vi "WS1050_RFFE_ST Scope Single Bit Measurement Debug Ver1.1.vi"(0 "RFFE PIC":refnum<visa-resource-name>="COM7", 1 "A3643A GPIB":refnum<visa-resource-name>="GPIB1::6::INSTR", 3 "LOT#":string="444AB", 4 "WAFER#":string="04", 5 "DUT SN":string="SN01", 7 "error in (no error)":errorcluster, 8 "Scope USB":refnum<visa-resource-name>="USB0::0x0699::0x0405::C010240::INSTR", 9 "GROUP":string, 12 "path":path=path "C:/Andy/WS1050/ST Test/Debug Ver1.1", 14 "Start":bool, 15 "Stop Loop":bool, 16 "Initilize RFFE ?":bool=TRUE, 17 "stop":bool, 20 "Scope \nSet Up":bool, 22 "Comment":string) -> (18 "ST Data Out":string[](array[string])=["824.709800E-9", "99.100000E+36", "14.400000E-3", "99.100000E+36", "687.070300E-9", "14.000000E-3", "991.902900E-9", "99.100000E+36", "30.800000E-3", "99.100000E+36", "729.561600E-9", "28.400000E-3", "794.023400E-9", "99.100000E+36", "66.000000E-3", "99.100000E+36", "698.320300E-9", "64.000000E-3", "677.011700E-9", "99.100000E+36", "172.000000E-3", "99.100000E+36", "781.972700E-9", "168.000000E-3", "1.047500E-6", "99.100000E+36", "252.000000E-3", "99.100000E+36", "806.324900E-9", "248.000000E-3", "1.166000E-6", "99.100000E+36", "384.000000E-3", "99.100000E+36", "800.507800E-9", "372.000000E-3", "3.559500E-6", "99.100000E+36", "536.000000E-3", "99.100000E+36", "804.648400E-9", "512.000000E-3", "2.976000E-6", "99.100000E+36", "664.000000E-3", "99.100000E+36", "794.980500E-9", "640.000000E-3", "1.596500E-6", "99.100000E+36", "792.000000E-3", "99.100000E+36", "835.996100E-9", "768.000000E-3", "3.144000E-6", "99.100000E+36", "912.000000E-3", "99.100000E+36", "849.980500E-9", "880.000000E-3", "1.416700E-6", "99.100000E+36", "1.000000E+0", "99.100000E+36", "864.023400E-9", "960.000000E-3", "1.295500E-6", "99.100000E+36", "1.060000E+0", "99.100000E+36", "858.515600E-9", "1.020000E+0", "1.204000E-6", "99.100000E+36", "1.080000E+0", "99.100000E+36", "934.023400E-9", "1.060000E+0", "1.336000E-6", "99.100000E+36", "1.140000E+0", "99.100000E+36", "1.063300E-6", "1.100000E+0", "1.338000E-6", "99.100000E+36", "1.160000E+0", "99.100000E+36", "1.149500E-6", "1.140000E+0", "1.280000E-6", "99.100000E+36", "1.200000E+0", "99.100000E+36", "1.149300E-6", "1.160000E+0", "1.380000E-6", "99.100000E+36", "1.200000E+0", "99.100000E+36", "1.173000E-6", "1.160000E+0", "1.408000E-6", "99.100000E+36", "1.220000E+0", "99.100000E+36", "1.194000E-6", "1.180000E+0", "1.215000E-6", "99.100000E+36", "70.000000E-3", "99.100000E+36", "1.033300E-6", "68.000000E-3", "2.179200E-6", "99.100000E+36", "170.000000E-3", "99.100000E+36", "1.326500E-6", "158.000000E-3", "1.427300E-6", "99.100000E+36", "316.000000E-3", "99.100000E+36", "1.133000E-6", "308.000000E-3", "1.174000E-6", "99.100000E+36", "680.000000E-3", "99.100000E+36", "915.325500E-9", "620.000000E-3", "1.356000E-6", "99.100000E+36", "920.000000E-3", "99.100000E+36", "1.156000E-6", "880.000000E-3", "1.310000E-6", "99.100000E+36", "960.000000E-3", "99.100000E+36", "1.476500E-6", "980.000000E-3", "1.482000E-6", "99.100000E+36", "1.080000E+0", "99.100000E+36", "1.526000E-6", "1.060000E+0", "1.539500E-6", "99.100000E+36", "1.140000E+0", "99.100000E+36", "1.666000E-6", "1.120000E+0", "1.567000E-6", "99.100000E+36", "1.160000E+0", "99.100000E+36", "1.768000E-6", "1.160000E+0", "1.520000E-6", "99.100000E+36", "1.200000E+0", "99.100000E+36", "1.804000E-6", "1.160000E+0", "1.515000E-6", "99.100000E+36", "1.200000E+0", "99.100000E+36", "1.898000E-6", "1.180000E+0", "1.498000E-6", "99.100000E+36", "1.220000E+0", "99.100000E+36", "1.858000E-6", "1.220000E+0", "1.449000E-6", "99.100000E+36", "1.220000E+0", "99.100000E+36", "1.870000E-6", "1.200000E+0", "1.458500E-6", "99.100000E+36", "1.220000E+0", "99.100000E+36", "1.860000E-6", "1.200000E+0", "1.428500E-6", "99.100000E+36", "1.220000E+0", "99.100000E+36", "1.870000E-6", "1.200000E+0", "1.350000E-6", "99.100000E+36", "1.200000E+0", "99.100000E+36", "1.918500E-6", "1.220000E+0", "1.468500E-6", "99.100000E+36", "1.220000E+0", "99.100000E+36", "1.938700E-6", "1.220000E+0", "1.390000E-6", "99.100000E+36", "1.200000E+0", "99.100000E+36", "1.917500E-6", "1.200000E+0", "634.023400E-9", "99.100000E+36", "46.000000E-3", "99.100000E+36", "1.470000E-6", "40.000000E-3", "1.126000E-6", "99.100000E+36", "84.000000E-3", "99.100000E+36", "1.137000E-6", "84.000000E-3", "1.103700E-6", "99.100000E+36", "238.000000E-3", "99.100000E+36", "1.126200E-6", "226.000000E-3", "1.091000E-6", "99.100000E+36", "512.000000E-3", "99.100000E+36", "1.010000E-6", "480.000000E-3", "3.414000E-6", "99.100000E+36", "760.000000E-3", "99.100000E+36", "949.980500E-9", "700.000000E-3", "1.376000E-6", "99.100000E+36", "940.000000E-3", "99.100000E+36", "1.268000E-6", "920.000000E-3", "1.268000E-6", "99.100000E+36", "1.020000E+0", "99.100000E+36", "1.278000E-6", "980.000000E-3", "1.294000E-6", "99.100000E+36", "1.060000E+0", "99.100000E+36", "1.334000E-6", "1.060000E+0", "1.488000E-6", "99.100000E+36", "1.160000E+0", "99.100000E+36", "1.448000E-6", "1.120000E+0", "1.515000E-6", "99.100000E+36", "1.200000E+0", "99.100000E+36", "1.534000E-6", "1.160000E+0", "1.516000E-6", "99.100000E+36", "1.240000E+0", "99.100000E+36", "1.628000E-6", "1.220000E+0", "1.602000E-6", "99.100000E+36", "1.280000E+0", "99.100000E+36", "1.557000E-6", "1.240000E+0", "1.610000E-6", "99.100000E+36", "1.300000E+0", "99.100000E+36", "1.637500E-6", "1.260000E+0", "1.580000E-6", "99.100000E+36", "1.300000E+0", "99.100000E+36", "1.724000E-6", "1.280000E+0", "1.611000E-6", "99.100000E+36", "1.320000E+0", "99.100000E+36", "1.722000E-6", "1.280000E+0", "1.611000E-6", "99.100000E+36", "1.320000E+0", "99.100000E+36", "1.770000E-6", "1.300000E+0", "1.608000E-6", "99.100000E+36", "1.320000E+0", "99.100000E+36", "1.780000E-6", "1.300000E+0", "1.601000E-6", "99.100000E+36", "1.320000E+0", "99.100000E+36", "1.795000E-6", "1.300000E+0"], 19 "ST Header Out":string[](array[string]), 21 "Status":string="Idle....", 27 "error out":errorcluster)   [LabVIEW 2012]
doc: "Ver1.0 has calculated and recorded both 60% and 95% of the AMP"
uses:
  <instrlib>/Tektronix DPO MSO 2000 4000 Series/Tektronix DPO MSO 2000 4000 Series.lvlib
panel:
  out "Filtered Signal":dbl[](graph)
  out "Signal":dbl[](graph)
  in  "% Amp_T3":dbl=0.95
  in  "% Amp_T2":dbl=0.9
  in  "Debug":bool
  in  "Loop Delay(s)":u32
  out "Index":i32
  in  "% Amp_T1":dbl=0.6
  out "Cmd Out":string
  in  "Bandwidth":u16(ring)=3 items=["FULL", "250 MHz", "150 MHz", "20 MHz"]
  out "Test Program Name":string=" WS1050 ST Scope SBM Debug Ver1.1"
  out "dt":dbl=1e-08
  in  "Timebase":dbl=0.0001
  in  "RFFE Action":i32(ring)=2 items=["-", "Charge Pump Off", "Charge Pump On", "-", "DVA OFF", "DVA ON", "Charge Pump to 40V", "Charge Pump to 35V", "Trim Code 26", "Trim Code 30", "Trim Code 32", "Trim Code 33", "Trim Code 42", "Trim Code 44", "Trim Code 46", "Trim Code 48", "Trim Code 49", "Trim Code 50", "All Drivers Off", "All Drivers On", "Reg1 On", "Reg2 On", "Reg3 On", "Reg4 On"]
  in  "RFFE Action":bool
  in  "Closing Cheetah function calls":i32(listbox)
  # "Updated based on Debug\n\n 1.  Updated WS1050 Extract Data From Scope_ST_CLK SubVI by adding another point   calculated based on 95% of Amp and 1 us for the CLK starts from 21st"
  # "Company:  WiSpry Inc\n20 Fairbanks Ste 198, Irvine\n\nAuthor:  Andy V Tran\nDate:  07/08/2015\nTP:  ST Scope Single Bit"
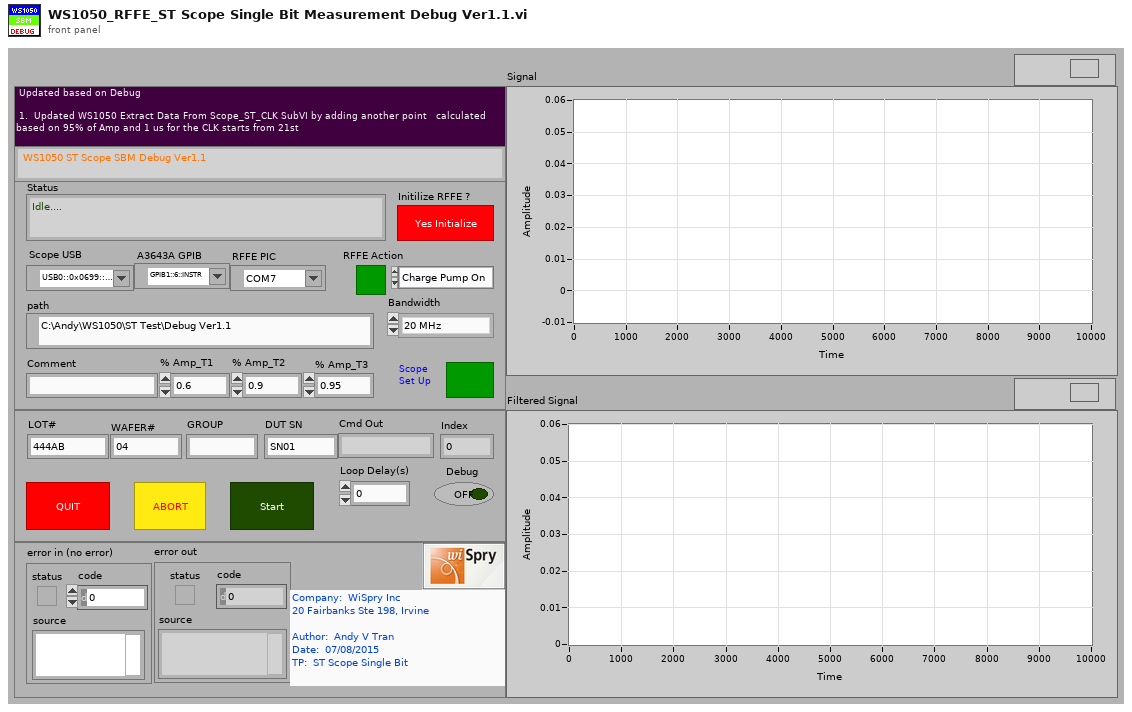
[diagram p1: front panel]
types:
  T1 = enum16{"open", "replace", "create", "open or create", "replace or create", "replace or create with confirmation"}
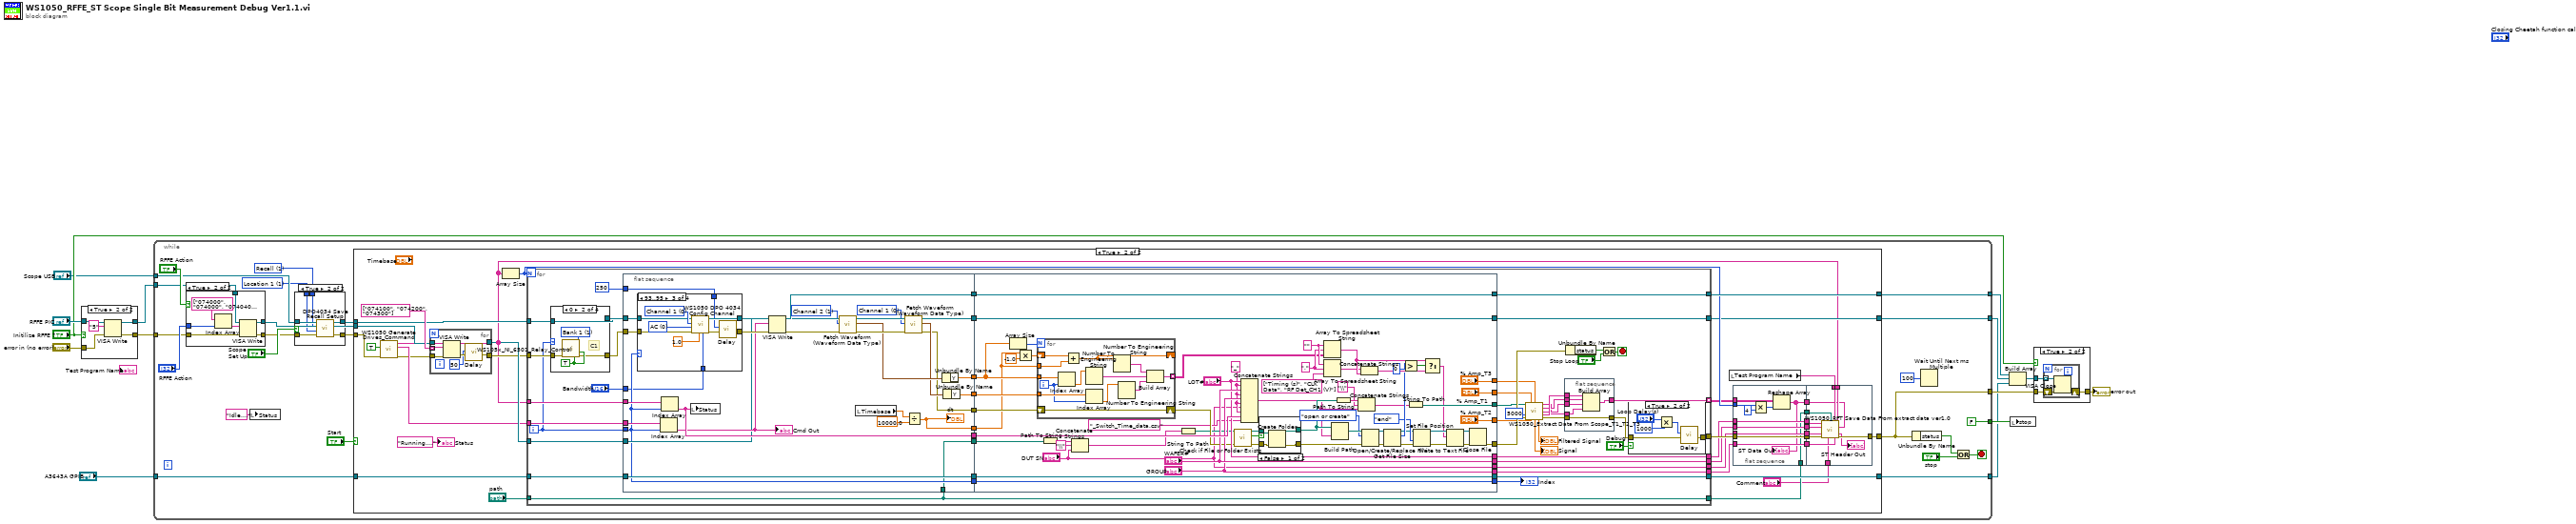
[diagram p0: block diagram]
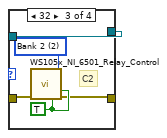
[diagram p7: hidden frame]
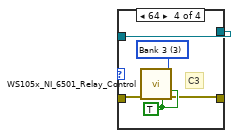
[diagram p8: hidden frame]
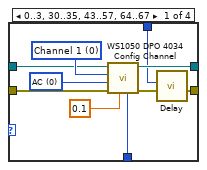
[diagram p9: hidden frame]
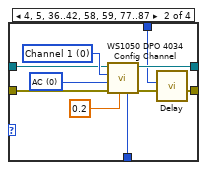
[diagram p10: hidden frame]
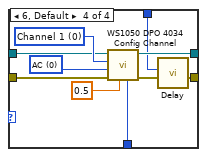
[diagram p11: hidden frame]
diagram:
  n1 = case shown="True" "Initilize RFFE ?" {
    tunnel: [w16 w18] -> w7
    tunnel: "error in (no error)" -> [w16 w19]
    tunnel: "RFFE PIC" -> [w15 w21]
    tunnel: [w15 w17] -> w9
    frame False {
    }
    frame True {
      n2 = VISA Write(VISA resource name=w21, write buffer="5", error in (no error)=w19) -> (VISA resource name out=w17:refnum<visa-resource-name>, error out=w18:errorcluster)  [unwired: 1 out]
    }
  }
  n3 = while {
    tunnel: [w37] -> w11
    tunnel: w7 -> [w30]
    tunnel: "A3643A GPIB" -> [w38]
    tunnel: [w36] -> w2
    tunnel: w9 -> [w29]
    tunnel: [w31] -> w4
    tunnel: [w27] -> w3
    tunnel: "Scope USB" -> [w26]
    tunnel: [FALSE ("stop")] -> w5
    stop <- w45 stop-if-true
    w23 = u16 1 items=["Location 1"=1, "Location 2"=2, "Location 3"=3, "Location 4"=4, "Location 5"=5, "Location 6"=6, "Location 7"=7, "Location 8"=8, "Location 9"=9, "Location 10"=10] ("Memory Location (1: Location 1)")
    w24 = u16 1 items=["Save", "Recall"] ("Operation (0: Save)")
    n4 = case shown="True" "RFFE Action" {
      tunnel: "RFFE Action" -> [_ w62]
      tunnel: w30 -> [w54 w60]
      tunnel: w29 -> [w55 w59]
      tunnel: [w55 w58] -> w28
      tunnel: [w54 w56] -> w25
      frame False {
      }
      frame True {
        n5 = Index Array(array=string[] ["074000", "074000", "074040", "", "074820", "074800", "074776", "07476F"], index=w62) -> (element=w57:string)
        n6 = VISA Write(VISA resource name=w59, write buffer=w57, error in (no error)=w60) -> (VISA resource name out=w58:refnum<visa-resource-name>, error out=w56:errorcluster)  [unwired: 1 out]
      }
    }
    n7 = local write "Status"("Idle...." ("Status")) -> ()
    n8 = case shown="True" "Scope \nSet Up" {
      tunnel: w25 -> [w47 w53]
      tunnel: [w47 w52] -> w33
      tunnel: w26 -> [w46 w51]
      tunnel: [w46 w50] -> w34
      tunnel: w24 -> [_ w49]
      tunnel: w23 -> [_ w48]
      frame False {
      }
      frame True {
        n9 = call "DPO4034 Save Recall Setup.vi"("error in (no error)"=w53, "Save/Recall"=w48, "Location"=w49, "VISA resource name"=w51) -> ("error out"=w52:errorcluster, "VISA resource name out"=w50:refnum<visa-resource-name>)  [unwired: 6 in]
      }
    }
    n10 = case shown="True" "Start" {
      tunnel: [w66 w83] -> w27
      tunnel: w34 -> [w66 w82]
      tunnel: w33 -> [w65 w71]
      tunnel: w38 -> [w64 w84]
      tunnel: [w64 w98] -> w36
      tunnel: [w65 w96] -> w37
      tunnel: [w63 w90] -> w31
      tunnel: w28 -> [w63 w86]
      frame False {
      }
      frame True {
        n11 = call "WS1050 Generate Drives_Command.vi"("error in (no error)"=w71, "ALL/UP-DN"=TRUE) -> ("error out"=w70:errorcluster, "Cmd"=w72:string[], "Driver Name"=w73:string[])  [unwired: 7 in]
        n12 = for {
          tunnel: w70 -> [w130]
          tunnel: w86 -> [w129]
          tunnel: [w128] -> w89
          tunnel: [w126] -> w88
          tunnel: string[] ["074100", "074200", "074300"] -> [w127] mode=indexing
          n13 = VISA Write(VISA resource name=w129, write buffer=w127, error in (no error)=w130) -> (VISA resource name out=w128:refnum<visa-resource-name>, error out=w125:errorcluster)  [unwired: 1 out]
          n14 = call "Delay.vi"("error in (no error)"=w125, "milliseconds to wait"=u32 50) -> ("error out"=w126:errorcluster)  [unwired: 9 in]
        }
        n15 = Array Size(array=w73) -> (size(s)=w85:i32)
        n16 = for {
          N: w85 -> [_]
          tunnel: [w143] -> w97
          tunnel: "path" -> [w148]
          tunnel: w84 -> [w172]
          tunnel: [w170] -> w98
          tunnel: w88 -> [w166]
          tunnel: w73 -> [w169]
          tunnel: w72 -> [w167]
          tunnel: [w163] -> w95
          tunnel: [w162] -> w94
          tunnel: [w161] -> w93
          tunnel: [w160] -> w92
          tunnel: w89 -> [w159]
          tunnel: [w157] -> w90
          tunnel: [w156] -> w83
          tunnel: w82 -> [w155]
          tunnel: [w148] -> w75
          tunnel: [w151] -> w69 mode=indexing
          i -> [w154]
          stop <- w178 stop-if-true
          n17 = case shown="0" w154 {
            tunnel: w166 -> [w193 w199 w204 w209]
            tunnel: [w193 w195 w200 w205] -> w165
            tunnel: w155 -> [w194 w196 w201 w206]
            tunnel: [w194 w196 w201 w206] -> w164
            frame 1, Default {
            }
            frame 0 {
              w197 = TRUE ("Relay_ 10")
              w198 = u16 1 items=["All Off", "Bank 1", "Bank 2", "Bank 3"] ("Ring")
              # "C1"
              n18 = call "WS105x_NI_6501_Relay_Control.vi"("Ring"=w198, "Relay_ 11"=w197, "error in (no error)"=w199, "Relay_ 10"=w197) -> ("error out"=w195:errorcluster)  [unwired: 2 in, 9 out]
            }
            frame 32 {
              w202 = TRUE ("Relay_ 10")
              w203 = u16 2 items=["All Off", "Bank 1", "Bank 2", "Bank 3"] ("Ring")
              # "C2"
              n19 = call "WS105x_NI_6501_Relay_Control.vi"("Ring"=w203, "Relay_ 11"=w202, "error in (no error)"=w204, "Relay_ 10"=w202) -> ("error out"=w200:errorcluster)  [unwired: 2 in, 9 out]
            }
            frame 64 {
              w207 = TRUE ("Relay_ 10")
              w208 = u16 3 items=["All Off", "Bank 1", "Bank 2", "Bank 3"] ("Ring")
              # "C3"
              n20 = call "WS105x_NI_6501_Relay_Control.vi"("Ring"=w208, "Relay_ 11"=w207, "error in (no error)"=w209, "Relay_ 10"=w207) -> ("error out"=w205:errorcluster)  [unwired: 2 in, 9 out]
            }
          }
          n21 = flat-sequence {
            tunnel: w154 -> [w221]
            tunnel: [w210] -> w177
            tunnel: [w211] -> w176
            tunnel: [w235] -> w175
            tunnel: [w234] -> w174
            tunnel: [w237] -> w173
            tunnel: w172 -> [w236]
            tunnel: [w236] -> w171
            tunnel: w165 -> [w232]
            tunnel: w164 -> [w231]
            tunnel: w169 -> [w229]
            tunnel: [w228] -> w168
            tunnel: w167 -> [w227]
            tunnel: w159 -> [w225]
            tunnel: [w224] -> w158
            tunnel: [w221] -> w150
            tunnel: w148 -> [w214]
            tunnel: [w214] -> w147
            tunnel: u32 250 ("Delay (ms)") -> [w213]
            tunnel: "Bandwidth" -> [w212]
            tunnel: [w338] -> w156
            tunnel: w177 -> [w338]
            tunnel: [w337] -> w153
            tunnel: w176 -> [w336]
            tunnel: w175 -> [w335]
            tunnel: w174 -> [w334]
            tunnel: w173 -> [w333]
            tunnel: w171 -> [w332]
            tunnel: [w332] -> w170
            tunnel: w168 -> [w331]
            tunnel: ["LOT#"] -> w163
            tunnel: ["WAFER#"] -> w162
            tunnel: ["GROUP"] -> w161
            tunnel: ["DUT SN"] -> w160
            tunnel: w158 -> [w330]
            tunnel: [w330] -> w157
            tunnel: [w326] -> w152
            tunnel: w150 -> [w325]
            tunnel: [w325] -> w149
            tunnel: w147 -> [w285]
            tunnel: ["% Amp_T1"] -> w146
            tunnel: ["% Amp_T2"] -> w141
            tunnel: ["% Amp_T3"] -> w137
            frame #0 {
              w216 = u16 0 items=["Channel 1", "Channel 2", "Channel 3", "Channel 4", "Math", "Reference 1", "Reference 2", "Reference 3", "Reference 4", "D0", "D1", "D2", "D3", "D4", "D5", "D6", "D7", "D8", "D9", "D10", "D11", "D12", "D13", "D14", "D15", "Amplitude", "Frequency", "Phase", "Normal", "Average", "Maximum Peak Hold", "Minimum Peak Hold"] ("Channel (0: Channel 1)")
              w217 = u16 1 items=["Channel 1", "Channel 2", "Channel 3", "Channel 4", "Math", "Reference 1", "Reference 2", "Reference 3", "Reference 4", "D0", "D1", "D2", "D3", "D4", "D5", "D6", "D7", "D8", "D9", "D10", "D11", "D12", "D13", "D14", "D15", "Amplitude", "Frequency", "Phase", "Normal", "Average", "Maximum Peak Hold", "Minimum Peak Hold"] ("Channel (0: Channel 1)")
              n22 = case shown="93..95" w221 {
                tunnel: w232 -> [w246 w256 w266 w276]
                tunnel: w231 -> [w245 w255 w265 w275]
                tunnel: [w244 w254 w264 w274] -> w230
                tunnel: w213 -> [w241 w251 w261 w269]
                tunnel: [w242 w252 w262 w272] -> w222
                tunnel: w212 -> [w239 w249 w259 w270]
                frame 0..3, 30..35, 43..57, 64..67 {
                  w248 = u16 0 items=["Channel 1", "Channel 2", "Channel 3", "Channel 4", "Math", "Reference 1", "Reference 2", "Reference 3", "Reference 4", "Bus 1", "Bus 2"] ("Channel (0: Channel 1)")
                  w247 = u16 0 items=["AC", "DC", "Ground"] ("Vertical Coupling (1: DC)")
                  n23 = call "WS1050 DPO 4034 Config Channel.vi"("Bandwidth (0: FULL)"=w239, "Vertical Range (10.0 V)"=0.1, "error in (no error)"=w246, "Vertical Coupling (1: DC)"=w247, "Channel (0: Channel 1)"=w248, "VISA resource name"=w245) -> ("error out"=w243:errorcluster, "VISA resource name out"=w242:refnum<visa-resource-name>)  [unwired: 4 in]
                  n24 = call "Delay.vi"("error in (no error)"=w243, "milliseconds to wait"=w241) -> ("error out"=w244:errorcluster)  [unwired: 9 in]
                }
                frame 4, 5, 36..42, 58, 59, 77..87 {
                  w258 = u16 0 items=["Channel 1", "Channel 2", "Channel 3", "Channel 4", "Math", "Reference 1", "Reference 2", "Reference 3", "Reference 4", "Bus 1", "Bus 2"] ("Channel (0: Channel 1)")
                  w257 = u16 0 items=["AC", "DC", "Ground"] ("Vertical Coupling (1: DC)")
                  n25 = call "WS1050 DPO 4034 Config Channel.vi"("Bandwidth (0: FULL)"=w249, "Vertical Range (10.0 V)"=0.2, "error in (no error)"=w256, "Vertical Coupling (1: DC)"=w257, "Channel (0: Channel 1)"=w258, "VISA resource name"=w255) -> ("error out"=w253:errorcluster, "VISA resource name out"=w252:refnum<visa-resource-name>)  [unwired: 4 in]
                  n26 = call "Delay.vi"("error in (no error)"=w253, "milliseconds to wait"=w251) -> ("error out"=w254:errorcluster)  [unwired: 9 in]
                }
                frame 93..95 {
                  w268 = u16 0 items=["Channel 1", "Channel 2", "Channel 3", "Channel 4", "Math", "Reference 1", "Reference 2", "Reference 3", "Reference 4", "Bus 1", "Bus 2"] ("Channel (0: Channel 1)")
                  w267 = u16 0 items=["AC", "DC", "Ground"] ("Vertical Coupling (1: DC)")
                  n27 = call "WS1050 DPO 4034 Config Channel.vi"("Bandwidth (0: FULL)"=w259, "Vertical Range (10.0 V)"=1.0, "error in (no error)"=w266, "Vertical Coupling (1: DC)"=w267, "Channel (0: Channel 1)"=w268, "VISA resource name"=w265) -> ("error out"=w263:errorcluster, "VISA resource name out"=w262:refnum<visa-resource-name>)  [unwired: 4 in]
                  n28 = call "Delay.vi"("error in (no error)"=w263, "milliseconds to wait"=w261) -> ("error out"=w264:errorcluster)  [unwired: 9 in]
                }
                frame 6, Default {
                  w278 = u16 0 items=["Channel 1", "Channel 2", "Channel 3", "Channel 4", "Math", "Reference 1", "Reference 2", "Reference 3", "Reference 4", "Bus 1", "Bus 2"] ("Channel (0: Channel 1)")
                  w277 = u16 0 items=["AC", "DC", "Ground"] ("Vertical Coupling (1: DC)")
                  n29 = call "WS1050 DPO 4034 Config Channel.vi"("Bandwidth (0: FULL)"=w270, "Vertical Range (10.0 V)"=0.5, "error in (no error)"=w276, "Vertical Coupling (1: DC)"=w277, "Channel (0: Channel 1)"=w278, "VISA resource name"=w275) -> ("error out"=w273:errorcluster, "VISA resource name out"=w272:refnum<visa-resource-name>)  [unwired: 4 in]
                  n30 = call "Delay.vi"("error in (no error)"=w273, "milliseconds to wait"=w269) -> ("error out"=w274:errorcluster)  [unwired: 9 in]
                }
              }
              n31 = Index Array(array=w227, index=w221) -> (element=w226:string)
              "Cmd Out" <- w226
              n32 = Index Array(array=w229, index=w221) -> (element=w228:string)
              n33 = local write "Status"(w228) -> ()
              n34 = VISA Write(VISA resource name=w225, write buffer=w226, error in (no error)=w230) -> (VISA resource name out=w224:refnum<visa-resource-name>, error out=w223:errorcluster)  [unwired: 1 out]
              n35 = call <instrlib>:"Fetch Waveform (Waveform Data Type).vi"("error in (no error)"=w223, "Channel (0: Channel 1)"=w217, "VISA resource name"=w222) -> ("error out"=w220:errorcluster, "Waveform Data"=w219:waveform(dbl), "VISA resource name out"=w218:refnum<visa-resource-name>)  [unwired: 6 in]
              n36 = local read "Timebase"() -> (w233:dbl)
              n37 = call <instrlib>:"Fetch Waveform (Waveform Data Type).vi"("error in (no error)"=w220, "Channel (0: Channel 1)"=w216, "VISA resource name"=w218) -> ("error out"=w211:errorcluster, "Waveform Data"=w215:waveform(dbl), "VISA resource name out"=w210:refnum<visa-resource-name>)  [unwired: 6 in]
              n38 = Divide(x=w233, y=10000.0) -> (x/y=w237:dbl)
              "dt" <- w237
              n39 = Unbundle By Name(w219) -> ("Y"=w235:dbl[])
              n40 = Unbundle By Name(w215) -> ("Y"=w234:dbl[])
            }
            frame #1 {
              w294 = "_" ("string")
              w321 = ""
              w320 = ","
              n41 = Array Size(array=w335) -> (size(s)=w299:i32)
              n42 = Multiply(x=w333, y=-1.0) -> (x*y=w297:dbl)
              n43 = for {
                N: w299 -> [_]
                tunnel: w335 -> [w346]
                tunnel: [w348] -> w298 mode=indexing
                shift-right: [w343] -> _
                shift-left: w297 -> [w344]
                tunnel: w334 -> [w341]
                tunnel: w333 -> [w339]
                shift-right: [w342] -> w300
                shift-left: w336 -> [w342]
                i -> [w340]
                n44 = Index Array(array=w346, index=w340) -> (element=w347:dbl)
                n45 = Add(x=w344, y=w339) -> (x+y=w343:dbl)
                n46 = Index Array(array=w341, index=w340) -> (element=w351:dbl)
                n47 = Number To Engineering String(4:w347) -> (0:w349:string)  [unwired: 3 in]
                n48 = Number To Engineering String(4:w343) -> (0:w345:string)  [unwired: 3 in]
                n49 = Number To Engineering String(4:w351) -> (0:w350:string)  [unwired: 3 in]
                n50 = Build Array(w345, w349, w350) -> (w348:string[])
              }
              n51 = Path To String(path=w285) -> (string=w293:string)
              n52 = Concatenate Strings(w293, "\\" ("string"), "DUT SN") -> (w292:string)
              n53 = String To Path(string=w292) -> (path=w291:path)
              n54 = call <vilib>:"Check if File or Folder Exists.vi"("error in (no error)"=w300, "path"=w291) -> ("error out"=w317:errorcluster, "file or folder exists?"=w319:bool, "dup path"=w316:path)  [unwired: 7 out]
              n55 = Concatenate Strings("LOT#", w294, "WAFER#", w294, "GROUP", w294, "DUT SN", w294, w331, "_Switch_Time_data.csv" ("string")) -> (w287:string)
              n56 = case shown="False" w319 {
                tunnel: w317 -> [w352 w357]
                tunnel: [w354 w357] -> w318
                tunnel: w316 -> [w355 w356]
                tunnel: [w353 w356] -> w290
                frame False {
                  n57 = Create Folder(path (use dialog)=w355, error in=w352) -> (created path=w353:path, error out=w354:errorcluster)  [unwired: 2 out]
                }
                frame True {
                }
              }
              n58 = Array To Spreadsheet String(delimiter (Tab)=w320, array=w298, 3:w321) -> (spreadsheet string=w322:string)
              n59 = Array To Spreadsheet String(delimiter (Tab)=w320, array=string[] ["Timing (s)", "CLK Data", "RF Det_CH1 (V)"] ("Array"), 3:w321) -> (spreadsheet string=w312:string)
              n60 = Build Path(base path=w290, name or relative path=w287) -> (appended path=w315:path)
              n61 = Path To String(path=w290) -> (string=w289:string)
              n62 = Concatenate Strings(w289, "\\" ("string"), w287) -> (w286:string)
              n63 = Concatenate Strings(w312, w322) -> (w313:string)
              n64 = Open/Create/Replace File(file path (use dialog)=w315, error in=w318, operation (0:open)=T1."open or create") -> (refnum out=w301:refnum<file>, error out=w305:errorcluster)  [unwired: 4 out]
              n65 = Get File Size(file=w301, error in=w305) -> (refnum out=w302:refnum<file>, size (in bytes)=w307:i64, 0:w303:errorcluster)
              n66 = Greater?(x=w307, y=i64 0) -> (0:w281:bool)
              n67 = String To Path(string=w286) -> (path=w326:path)
              n68 = Set File Position(refnum=w302, from (0:start)=enum16{"start", "end", "current"}."end", error in=w303) -> (refnum out=w324:refnum<file>, error out=w304:errorcluster)  [unwired: 1 out]
              n69 = Select(t=w322, s=w281, f=w313) -> (s? t:f=w323:string)
              n70 = Write to Text File(file (use dialog)=w324, text=w323, error in=w304) -> (refnum out=w310:refnum<file>, error out=w309:errorcluster)  [unwired: 2 out]
              n71 = Close File(refnum=w310, error in=w309) -> (error out=w337:errorcluster)  [unwired: 1 out]
            }
          }
          n72 = call "WS1050_Extract Data From Scope_T1_T2_T3.vi"("file path"=w152, "60% Amp"=w146, "95% Amp"=w137, "Set Point for AMP"=5000 ("End point"), "error in (no error)"=w153, "90% Amp"=w141) -> ("Amp(mv)"=w133:string, "T2(us)"=w135:string, "T3(us)"=w134:string, "T1(us)"=w136:string, "Signal"=→"Signal":dbl[], "Filtered Signal"=→"Filtered Signal":dbl[], "error out"=w140:errorcluster)  [unwired: 2 in, 1 out]
          n73 = flat-sequence {
            tunnel: [w186] -> w151
            tunnel: w140 -> [w185]
            tunnel: [w185] -> w139
            tunnel: w136 -> [w184]
            tunnel: w135 -> [w183]
            tunnel: w134 -> [w182]
            tunnel: w133 -> [w181]
            frame #0 {
              n74 = Build Array(w184, w183, w182, w181) -> (w186:string[])
            }
          }
          n75 = Unbundle By Name(w153) -> ("status"=w180:bool)
          n76 = Or(x=w180, y="Stop Loop") -> (x .or. y?=w178:bool)
          n77 = case shown="True" "Debug" {
            tunnel: [w187 w192] -> w143
            tunnel: w139 -> [w187 w191]
            frame False {
            }
            frame True {
              n78 = Multiply(x="Loop Delay(s)", y=u32 1000) -> (x*y=w188:u32)
              n79 = call "Delay.vi"("error in (no error)"=w191, "milliseconds to wait"=w188) -> ("error out"=w192:errorcluster)  [unwired: 9 in]
            }
          }
          "Index" <- w149
        }
        n80 = local read "Test Program Name"() -> (w91:string)
        n81 = flat-sequence {
          tunnel: w85 -> [w101]
          tunnel: w92 -> [w107]
          tunnel: w93 -> [w108]
          tunnel: w94 -> [w109]
          tunnel: w95 -> [w110]
          tunnel: w97 -> [w111]
          tunnel: [w111] -> w81
          tunnel: [w110] -> w80
          tunnel: [w109] -> w79
          tunnel: [w108] -> w78
          tunnel: [w107] -> w77
          tunnel: [w106] -> w76
          tunnel: w69 -> [w105]
          tunnel: w75 -> [w104]
          tunnel: [w104] -> w74
          tunnel: [w122] -> w96
          tunnel: w91 -> [w117]
          tunnel: w73 -> [w116]
          tunnel: w81 -> [w123]
          tunnel: w80 -> [w121]
          tunnel: w79 -> [w120]
          tunnel: w78 -> [w119]
          tunnel: w77 -> [w118]
          tunnel: w76 -> [w114]
          tunnel: w74 -> [w113]
          tunnel: "Comment" -> [w112]
          frame #0 {
            n82 = Multiply(x=w101, y=4) -> (x*y=w103:i32)
            n83 = Reshape Array(w105, w103) -> (w106:string[])
            "ST Data Out" <- w106
          }
          frame #1 {
            n84 = call "WS1050_RFT Save Data From extract data ver1.0.vi"("Lot#"=w121, "RFT Path"=w113, "Test Program Name"=w117, "Driver Name"=w116, "Wafer#"=w120, "RFT"=w114, "SN#"=w118, "error in (no error)"=w123, "Comment"=w112, "Group#"=w119) -> ("ST Header Out"=→"ST Header Out":string[], "error out"=w122:errorcluster)  [unwired: 4 in]
          }
        }
        "Status" <- "Running...." ("Status")
      }
    }
    n85 = Unbundle By Name(w37) -> ("status"=w44:bool)
    n86 = Wait Until Next ms Multiple(millisecond multiple=u32 100) -> ()  [unwired: 1 out]
    n87 = Or(x=w44, y="stop") -> (x .or. y?=w45:bool)
  }
  n88 = Build Array(w4, w3, w2) -> (w1:refnum<visa-resource-name>[])
  n89 = local write "stop"(w5) -> ()
  n90 = case shown="True" "Initilize RFFE ?" {
    tunnel: w11 -> [w358 w361]
    tunnel: [w358 w360] -> w13
    tunnel: w1 -> [_ w359]
    frame False {
    }
    frame True {
      n91 = for {
        tunnel: w359 -> [w362] mode=indexing
        shift-right: [w363] -> w360
        shift-left: w361 -> [w364]
        n92 = VISA Close(VISA resource name=w362, error in (no error)=w364) -> (error out=w363:errorcluster)
      }
    }
  }
  "error out" <- w13
